vi "Logout Role.vi"(8 "error in (no error)":errorcluster, 11 "Roles API in":refnum<class "Roles API.lvclass">) -> (0 "error out":errorcluster, 3 "Roles API out":refnum<class "Roles API.lvclass">)   [LabVIEW 2020, in "Volatus.lvlib" / "Roles API.lvclass"]
uses:
  Roles API.lvclass
  Roles API.lvclass/Roles API.ctl
  MessageQ/MessageQ.lvclass
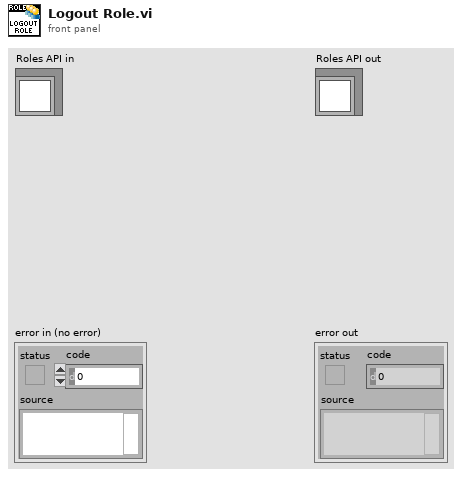
[diagram p1: front panel]
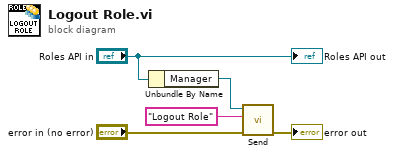
[diagram p0: block diagram]
diagram:
  n1 = Unbundle By Name("Roles API in") -> ("Manager"=w4:refnum<class "MessageQ.lvclass">)
  n2 = call "Send.vi"("error in (no error)"="error in (no error)", "ID"="Logout Role", "MessageQ in"=w4) -> ("error out"=→"error out":errorcluster)  [unwired: 7 in, 1 out]
  "Roles API out" <- "Roles API in"
